vi "Shared_Close.vi"(9 "Reset?":bool, 10 "Driver":T1(ring), 11 "Semiconductor Module Context":T2) -> (0 "error out":errorcluster)   [LabVIEW 2020, in "Shared.lvlib"]
doc: "Close instruments sessions"
uses:
  Shared.lvlib
  <vilib>/NI_TestStand_SemiconductorModule/NI_TestStand_Semiconductor_Module.lvlibp/PinMap/General/SemiconductorModuleContext.ctl
  <vilib>/NI_TestStand_SemiconductorModule/NI_TestStand_Semiconductor_Module.lvlibp
  ResourceHandling/ResourceHandling.lvlib
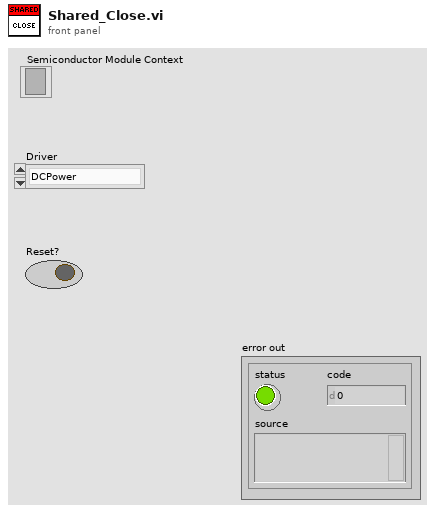
[diagram p1: front panel]
types:
  T1 = enum16{"DCPower", "SCOPE", "FGEN", "Relays", "PPMU"}
  T2 = typedef "NI_TestStand_Semiconductor_Module.lvlibp/SemiconductorModuleContext.ctl" = refnum<k7>
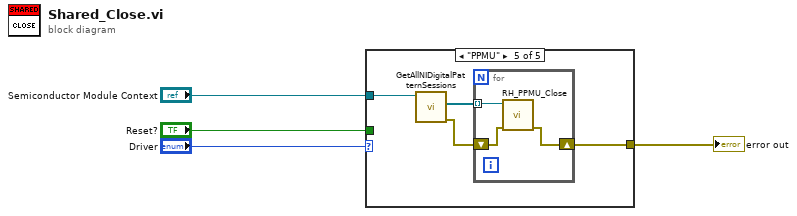
[diagram p0: block diagram]
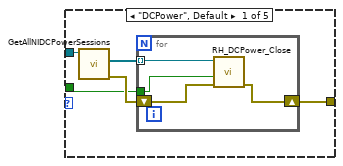
[diagram p2: hidden frame]
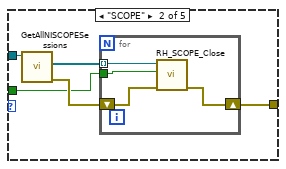
[diagram p3: hidden frame]
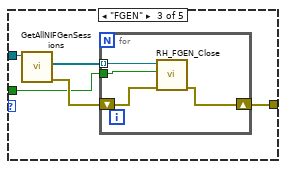
[diagram p4: hidden frame]
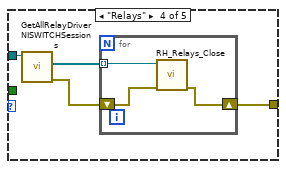
[diagram p5: hidden frame]
diagram:
  n1 = case shown="\"PPMU\"" "Driver" {
    tunnel: "Semiconductor Module Context" -> [w9 w18 w27 w35 w42]
    tunnel: [w6 w15 w24 w32 w39] -> w3
    tunnel: "Reset?" -> [w5 w14 w23 _ _]
    frame "DCPower", Default {
      n2 = call <vilib>:"GetAllNIDCPowerSessions.vi"("Semiconductor Module Context"=w9) -> ("error out"=w8:errorcluster, "Instrument Sessions"=w7:refnum<k15>[])  [unwired: 8 in, 1 out]
      n3 = for {
        tunnel: w7 -> [w12] mode=indexing
        shift-right: [w11] -> w6
        shift-left: w8 -> [w13]
        tunnel: w5 -> [w10]
        n4 = call "RH_DCPower_Close.vi"("error in (no error)"=w13, "Reset?"=w10, "DCPower Session In"=w12) -> ("error out"=w11:errorcluster)  [unwired: 8 in]
      }
    }
    frame "SCOPE" {
      n5 = call <vilib>:"GetAllNISCOPESessions.vi"("Semiconductor Module Context"=w18) -> ("error out"=w17:errorcluster, "Instrument Sessions"=w16:refnum<k15>[])  [unwired: 8 in, 1 out]
      n6 = for {
        tunnel: w16 -> [w21] mode=indexing
        shift-right: [w20] -> w15
        shift-left: w17 -> [w22]
        tunnel: w14 -> [w19]
        n7 = call "RH_SCOPE_Close.vi"("error in (no error)"=w22, "Reset?"=w19, "SCOPE Session In"=w21) -> ("error out"=w20:errorcluster)  [unwired: 8 in]
      }
    }
    frame "FGEN" {
      n8 = call <vilib>:"GetAllNIFGenSessions.vi"("Semiconductor Module Context"=w27) -> ("error out"=w26:errorcluster, "Instrument Sessions"=w25:refnum<k15>[])  [unwired: 8 in, 1 out]
      n9 = for {
        tunnel: w25 -> [w30] mode=indexing
        shift-right: [w29] -> w24
        shift-left: w26 -> [w31]
        tunnel: w23 -> [w28]
        n10 = call "RH_FGEN_Close.vi"("error in"=w31, "Reset"=w28, "FGEN Session In"=w30) -> ("error out"=w29:errorcluster)  [unwired: 8 in]
      }
    }
    frame "Relays" {
      n11 = call <vilib>:"GetAllRelayDriverNISWITCHSessions.vi"("Semiconductor Module Context"=w35) -> ("error out"=w34:errorcluster, "NI-SWITCH Sessions"=w33:refnum<k15>[])  [unwired: 8 in, 1 out]
      n12 = for {
        tunnel: w33 -> [w37] mode=indexing
        shift-right: [w36] -> w32
        shift-left: w34 -> [w38]
        n13 = call "RH_Relays_Close.vi"("error in"=w38, "Relays Session In"=w37) -> ("error out"=w36:errorcluster)  [unwired: 9 in]
      }
    }
    frame "PPMU" {
      n14 = call <vilib>:"GetAllNIDigitalPatternSessions.vi"("Semiconductor Module Context"=w42) -> ("error out"=w40:errorcluster, "Instrument Sessions"=w41:refnum<k15>[])  [unwired: 8 in, 1 out]
      n15 = for {
        tunnel: w41 -> [w45] mode=indexing
        shift-right: [w43] -> w39
        shift-left: w40 -> [w44]
        n16 = call "RH_PPMU_Close.vi"("error in"=w44, "PPMU Session In"=w45) -> ("error out"=w43:errorcluster)  [unwired: 9 in]
      }
    }
  }
  "error out" <- w3
